vi "SetControlSize.vi"(0 "时频域1":refnum<vi>, 1 "Choose1":refnum<vi>, 2 "录波开始时间":refnum<vi>, 3 "已录波":refnum<vi>, 4 "录波文件大小":refnum<vi>, 5 "Graph1":refnum<vi>, 6 "XYGraph":refnum<vi>, 7 "Pane Refnum":refnum<vi>, 8 "Mode":refnum<vi>, 9 "Graph2":refnum<vi>, 10 "录波？":refnum<vi>, 11 "时频域2":refnum<vi>, 12 "Choose2":refnum<vi>) -> ()   [LabVIEW 2014]
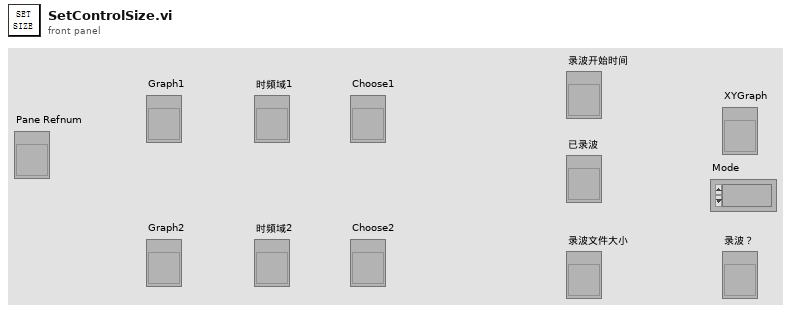
[diagram p1: front panel]
types:
  T1 = typedef "LVRectTypeDef.ctl" = cluster{"Left":i16, "Top":i16, "Right":i16, "Bottom":i16}
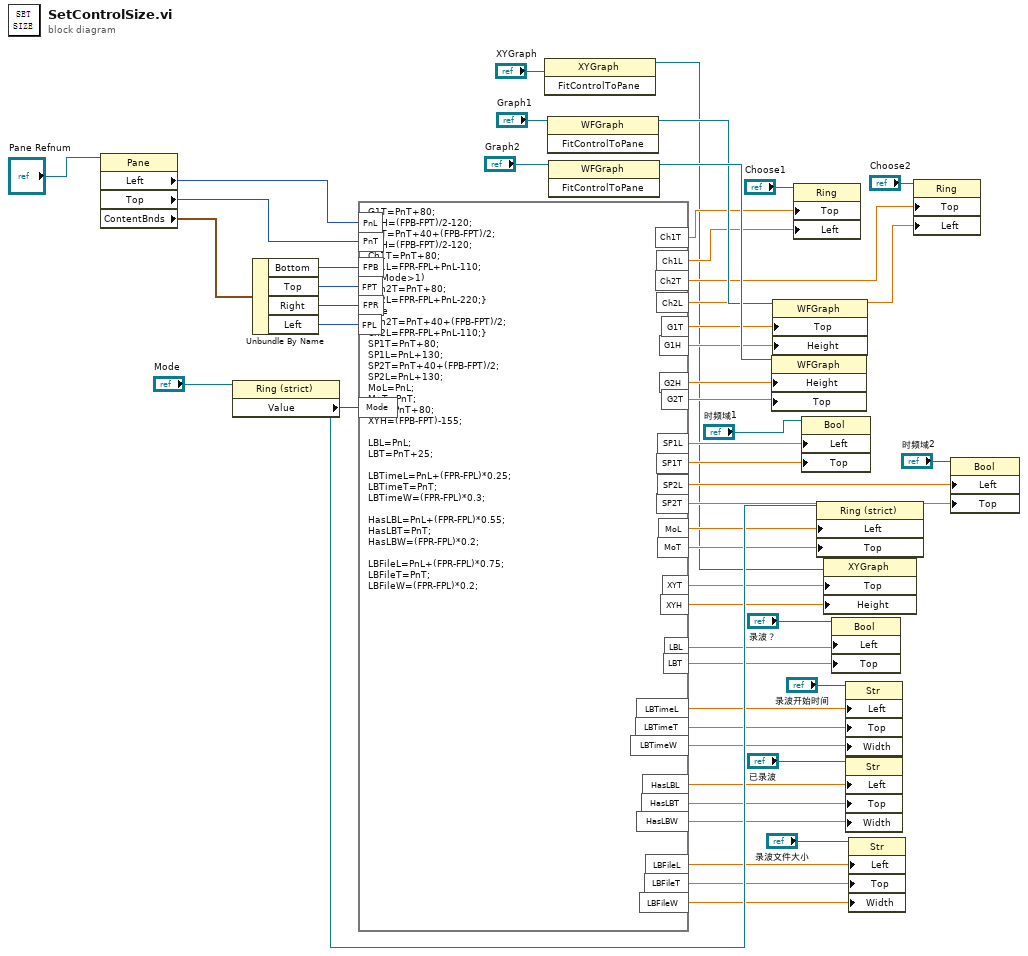
[diagram p0: block diagram]
diagram:
  n1 = property class="Pane"(reference="Pane Refnum") -> ("Left"=w2:i32, "Top"=w1:i32, "ContentBnds"=w46:T1)  [unwired: 1 in, 2 out]
  n2 = property class="Ring (strict)"(reference="Mode") -> (reference out=w25:refnum<vi>, "Value"=w26:u16)  [unwired: 1 in, 1 out]
  n3 = Unbundle By Name(w46) -> ("Bottom"=w45:i16, "Top"=w44:i16, "Right"=w43:i16, "Left"=w42:i16)
  n4 = formula code="G1T=PnT+80;\nG1H=(FPB-FPT)/2-120;\nG2T=PnT+40+(FPB-FPT)/2;\nG2H=(FPB-FPT)/2-120;\nCh1T=PnT+80;\nCh1L=FPR-FPL+PnL-110;\nif (Mode>1)\n{Ch2T=PnT+80;\nCh2L=FPR-FPL+PnL-220;}\nelse\n{Ch2T=PnT+40+(FPB-FPT)/2;\nCh2L=FPR-FPL+PnL-110;}\nSP1T=PnT+80;\nSP1L=PnL+130;\nSP2T=PnT+40+(FPB-FPT)/2;\nSP2L=PnL+130;\nMoL=PnL;\nMoT=PnT;\nXYT=PnT+80;\nXYH=(FPB-FPT)-155;\n\nLBL=PnL;\nLBT=PnT+25;\n\nLBTimeL=PnL+(FPR-FPL)*0.25;\nLBTimeT=PnT;\nLBTimeW=(FPR-FPL)*0.3;\n\nHasLBL=PnL+(FPR-FPL)*0.55;\nHasLBT=PnT;\nHasLBW=(FPR-FPL)*0.2;\n\nLBFileL=PnL+(FPR-FPL)*0.75;\nLBFileT=PnT;\nLBFileW=(FPR-FPL)*0.2;"("FPB"=w45, "FPT"=w44, "FPR"=w43, "FPL"=w42, "PnT"=w1, "PnL"=w2, "Mode"=w26) -> ("G1H"=w39:dbl, "G2H"=w40:dbl, "G1T"=w38:dbl, "G2T"=w41:dbl, "Ch1T"=w37:dbl, "Ch1L"=w36:dbl, "Ch2T"=w35:dbl, "Ch2L"=w34:dbl, "SP1T"=w30:dbl, "SP1L"=w31:dbl, "SP2T"=w29:dbl, "SP2L"=w28:dbl, "MoL"=w24:dbl, "MoT"=w23:dbl, "XYT"=w22:dbl, "XYH"=w21:dbl, "LBL"=w17:dbl, "LBT"=w16:dbl, "LBTimeL"=w14:dbl, "LBTimeT"=w13:dbl, "LBFileL"=w8:dbl, "LBFileT"=w7:dbl, "HasLBL"=w11:dbl, "HasLBT"=w10:dbl, "LBTimeW"=w6:dbl, "HasLBW"=w5:dbl, "LBFileW"=w4:dbl)
  n5 = invoke class="XYGraph" method="FitControlToPane"(reference="XYGraph") -> (reference out=w19:refnum<vi>)  [unwired: 2 in, 2 out]
  n6 = invoke class="WFGraph" method="FitControlToPane"(reference="Graph1") -> (reference out=w51:refnum<vi>)  [unwired: 2 in, 2 out]
  n7 = invoke class="WFGraph" method="FitControlToPane"(reference="Graph2") -> (reference out=w52:refnum<vi>)  [unwired: 2 in, 2 out]
  n8 = property class="WFGraph"(reference=w52, "Height"=w40, "Top"=w41) -> ()  [unwired: 1 in, 2 out]
  n9 = property class="WFGraph"(reference=w51, "Top"=w38, "Height"=w39) -> ()  [unwired: 1 in, 2 out]
  n10 = property class="Ring"(reference="Choose1", "Top"=w37, "Left"=w36) -> ()  [unwired: 1 in, 2 out]
  n11 = property class="Bool"(reference="时频域1", "Left"=w31, "Top"=w30) -> ()  [unwired: 1 in, 2 out]
  n12 = property class="Ring (strict)"(reference=w25, "Left"=w24, "Top"=w23) -> ()  [unwired: 1 in, 2 out]
  n13 = property class="XYGraph"(reference=w19, "Top"=w22, "Height"=w21) -> ()  [unwired: 1 in, 2 out]
  n14 = property class="Bool"(reference="录波？", "Left"=w17, "Top"=w16) -> ()  [unwired: 1 in, 2 out]
  n15 = property class="Str"(reference="录波开始时间", "Left"=w14, "Top"=w13, "Width"=w6) -> ()  [unwired: 1 in, 2 out]
  n16 = property class="Str"(reference="已录波", "Left"=w11, "Top"=w10, "Width"=w5) -> ()  [unwired: 1 in, 2 out]
  n17 = property class="Str"(reference="录波文件大小", "Left"=w8, "Top"=w7, "Width"=w4) -> ()  [unwired: 1 in, 2 out]
  n18 = property class="Ring"(reference="Choose2", "Top"=w35, "Left"=w34) -> ()  [unwired: 1 in, 2 out]
  n19 = property class="Bool"(reference="时频域2", "Left"=w28, "Top"=w29) -> ()  [unwired: 1 in, 2 out]
